vi "Create.vi"(8 "error in (no error)":errorcluster, 11 "Database Manager":refnum<class "Database Manager.lvclass">) -> (0 "error out":errorcluster, 3 "Dataset out":refnum<class "Dataset.lvclass">)   [LabVIEW 2019, in "HierDAL Library.lvlib" / "Database.lvlib" / "Repositories.lvlib" / "Dataset.lvclass"]
uses:
  Dataset.lvclass
  Database Manager Class/Database Manager.lvclass
  Dataset.lvclass/Dataset.ctl
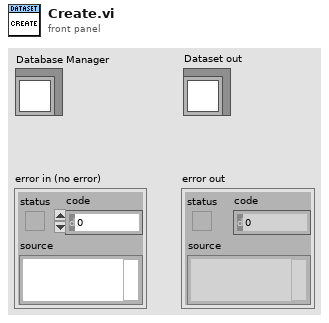
[diagram p1: front panel]
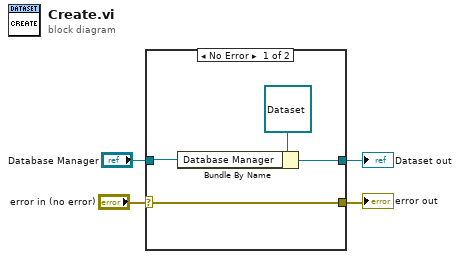
[diagram p0: block diagram]
diagram:
  n1 = case shown="No Error" "error in (no error)" {
    selector: "error in (no error)" -> [w8 w9]
    tunnel: [w8 w9] -> w1
    tunnel: [w6 _] -> w2
    tunnel: "Database Manager" -> [w7 _]
    frame No Error {
      n2 = Bundle By Name(cluster=refnum<class "Dataset.lvclass"> refnum ("Parent Child out"), "Database Manager"=w7) -> (w6:refnum<class "Dataset.lvclass">)
    }
    frame Error {
    }
  }
  "error out" <- w1
  "Dataset out" <- w2
